vi "Logger_QueueRef.vi"(8 "error in (no error)":errorcluster caption="错误输入（无错误）", 11 "Logger 输入":refnum<class "Logger.lvclass">) -> (0 "error out":errorcluster caption="错误输出", 3 "Logger 输出":refnum<class "Logger.lvclass">)   [LabVIEW 2019, in "Logger.lvclass"]
uses:
  <userlib>/Logger/Logger.lvclass
  <userlib>/Logger/Ctls/LoggerMessage.ctl
  <userlib>/Logger/Logger.lvclass/Logger.ctl
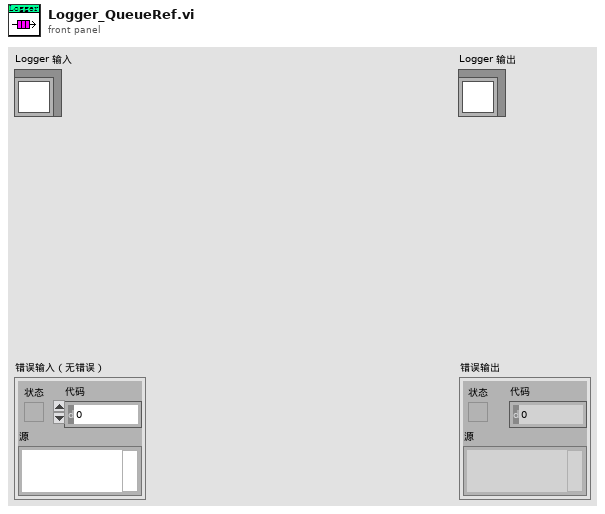
[diagram p1: front panel]
types:
  T1 = typedef "Logger.lvclass/LoggerMessage.ctl" = cluster{"LoggerKind":enum16{"软件上传日志", "软件其他日志", "软件错误日志", "软件监控日志"}, "LoggerMessage":string, "LoggerCode":i32, "LoggerCallChain":string, "LoggerTime":string}
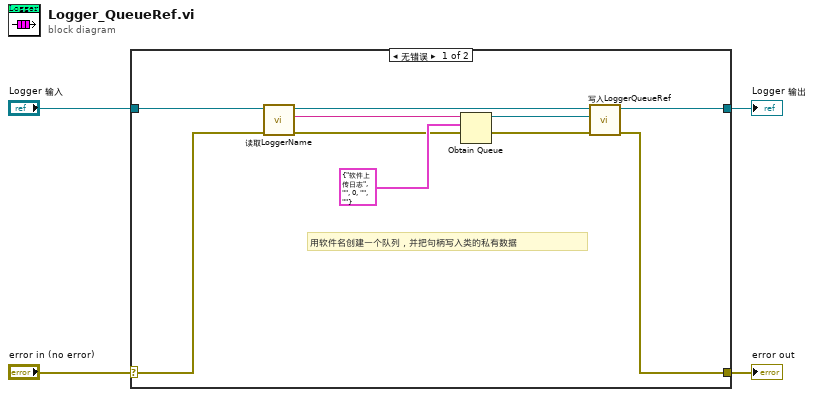
[diagram p0: block diagram]
diagram:
  n1 = case shown="无错误" "error in (no error)" {
    selector: "error in (no error)" -> [w6 w16]
    tunnel: [w7 w16] -> w3
    tunnel: [w10 w15] -> w1
    tunnel: "Logger 输入" -> [w14 w15]
    frame No Error {
      # "用软件名创建一个队列，并把句柄写入类的私有数据"
      n2 = call "读取LoggerName.vi"("error in (no error)"=w6, "Logger输入"=w14) -> ("error out"=w5:errorcluster, "LoggerName"=w12:string, "Logger输出"=w13:refnum<class "Logger.lvclass">)  [unwired: 7 in]
      n3 = Obtain Queue(name (unnamed)=w12, element data type=T1 {"LoggerKind"=enum."软件上传日志", "LoggerMessage"="", "LoggerCode"=0, "LoggerCallChain"="", "LoggerTime"=""} ("Logger"), error in (no error)=w5) -> (queue out=w9:refnum<queue>, error out=w8:errorcluster)  [unwired: 2 in, 1 out]
      n4 = call "写入LoggerQueueRef.vi"("error in (no error)"=w8, "LoggerQueueRef"=w9, "Logger输入"=w13) -> ("error out"=w7:errorcluster, "Logger输出"=w10:refnum<class "Logger.lvclass">)  [unwired: 7 in]
    }
    frame Error {
    }
  }
  "error out" <- w3
  "Logger 输出" <- w1
